vi "Print_Messages.vi"() -> ()   [LabVIEW 2012]
uses:
  Globals/Status_Error_Messages.vi
panel:
  out "String":string
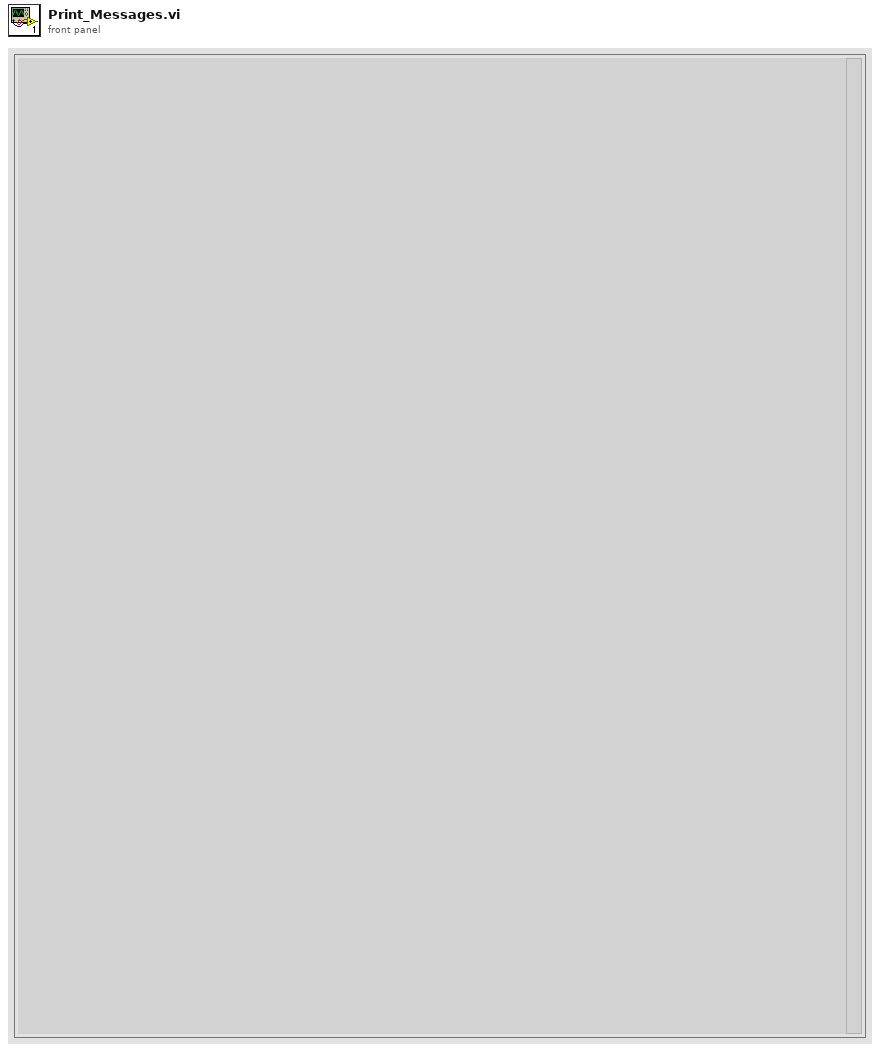
[diagram p1: front panel]
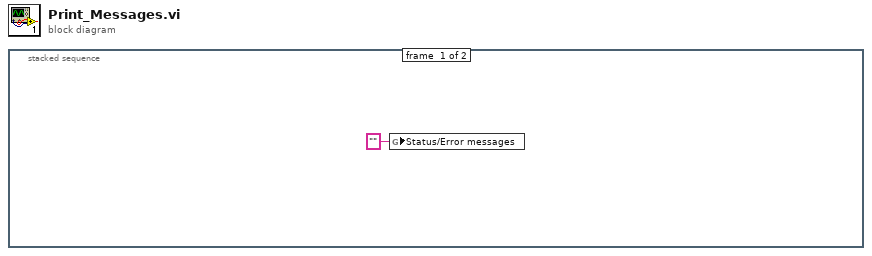
[diagram p0: block diagram]
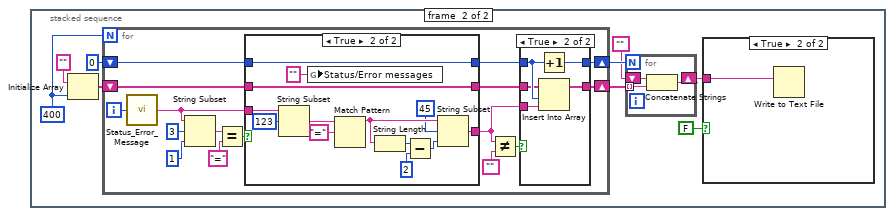
[diagram p2: hidden frame]
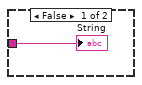
[diagram p3: hidden frame]
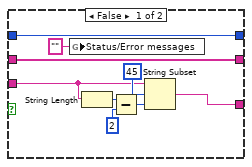
[diagram p4: hidden frame]
diagram:
  n1 = stacked-sequence {
    frame #0 {
      n2 = global write "Status_Error_Messages.vi" "Status/Error messages"("" ("Status/Error messages")) -> ()
    }
    frame #1 {
      w4 = 400 ("dimension size")
      n3 = Initialize Array("" ("element"), w4) -> (w9:string[])
      n4 = for {
        N: w4 -> [_]
        shift-right: [w31] -> w8
        shift-left: 0 -> [w18]
        shift-right: [w26] -> w7
        shift-left: w9 -> [w19]
        i -> [w30]
        n5 = call "Status_Error_Message.vi"("Message number"=w30) -> ("Status/Error string"=w23:string)
        n6 = String Subset(string=w23, offset (0)=3, length (rest)=1 ("length (rest)")) -> (substring=w22:string)
        n7 = Equal?(x=w22, y="=") -> (x = y?=w24:bool)
        n8 = case shown="True" w24 {
          tunnel: [w39 w49] -> w21
          tunnel: w23 -> [w38 w52]
          tunnel: w19 -> [w34 w43]
          tunnel: [w34 w43] -> w17
          tunnel: w18 -> [w33 w42]
          tunnel: [w33 w42] -> w16
          frame False {
            n9 = global write "Status_Error_Messages.vi" "Status/Error messages"("" ("Status/Error messages")) -> ()
            n10 = String Length(string=w38) -> (length=w37:i32)
            n11 = Subtract(x=w37, y=2) -> (x-y=w36:i32)
            n12 = String Subset(string=w38, offset (0)=45, length (rest)=w36) -> (substring=w39:string)
          }
          frame True {
            n13 = String Subset(string=w52, offset (0)=123) -> (substring=w51:string)  [unwired: 1 in]
            n14 = global write "Status_Error_Messages.vi" "Status/Error messages"("" ("Status/Error messages")) -> ()
            n15 = Match Pattern(string=w51, regular expression="=") -> (before substring=w48:string)  [unwired: 1 in, 3 out]
            n16 = String Length(string=w48) -> (length=w46:i32)
            n17 = Subtract(x=w46, y=2) -> (x-y=w47:i32)
            n18 = String Subset(string=w48, offset (0)=45, length (rest)=w47) -> (substring=w49:string)
          }
        }
        n19 = Not Equal?(x=w21, y="") -> (x != y?=w20:bool)
        n20 = case shown="True" w20 {
          tunnel: w16 -> [w55 w58]
          tunnel: [w55 w60] -> w31
          tunnel: w17 -> [w54 w57]
          tunnel: [w54 w59] -> w26
          tunnel: w21 -> [_ w56]
          frame False {
          }
          frame True {
            n21 = Increment(x=w58) -> (x+1=w60:i32)
            n22 = Insert Into Array(array=w57, index=w58, new element=w56) -> (w59:string[])
          }
        }
      }
      n23 = for {
        N: w8 -> [_]
        tunnel: w7 -> [w13] mode=indexing
        shift-right: [w15] -> w5
        shift-left: "" -> [w14]
        n24 = Concatenate Strings(w14, w13) -> (w15:string)
      }
      n25 = case shown="True" FALSE {
        tunnel: w5 -> [w11 w12]
        frame False {
          "String" <- w11
        }
        frame True {
          n26 = Write to Text File(text=w12) -> ()  [unwired: 3 in, 3 out]
        }
      }
    }
  }
